vi "Write.vi"(8 "error in (no error)":errorcluster, 9 "Variant":variant, 10 "String":string, 11 "UDP in":refnum<class "UDP.lvclass">) -> (0 "error out":errorcluster, 3 "UDP out":refnum<class "UDP.lvclass">)   [LabVIEW 2019, in "Protocols.lvlib" / "UDP.lvclass"]
uses:
  UDP.lvclass
  UDP.lvclass/UDP.ctl
  Data Access/Read Target Port.vi
  Data Access/Read Target IP Address.vi
  Data Access/Read UDP Ref.vi
  Data Access/Write UDP Ref.vi
  <vilib>/Utility/error.llb/Clear Errors.vi
  Protocol Parent/Protocol Parent.lvclass
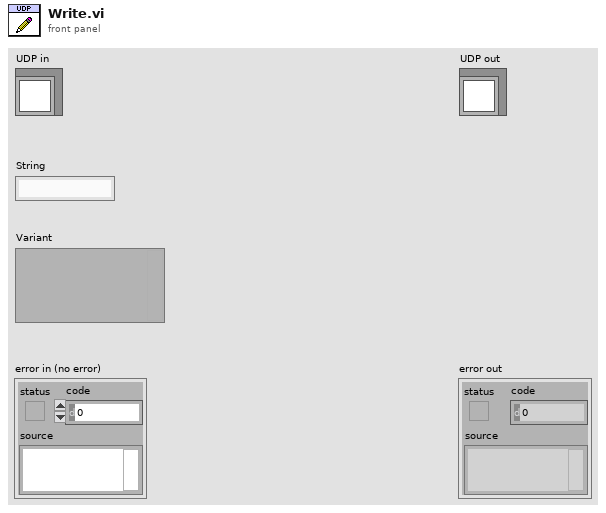
[diagram p1: front panel]
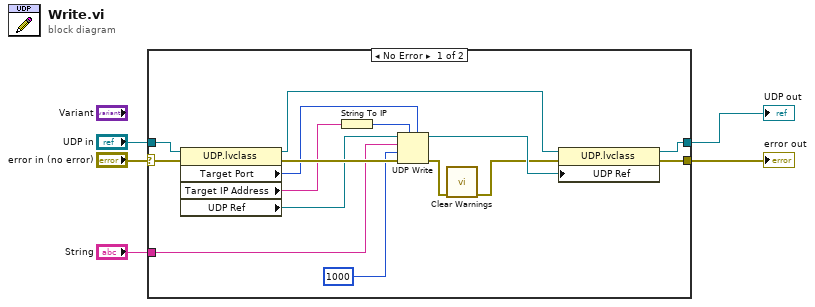
[diagram p0: block diagram]
diagram:
  n1 = case shown="No Error" "error in (no error)" {
    selector: "error in (no error)" -> [w13 w22]
    tunnel: "UDP in" -> [w19 w21]
    tunnel: [w16 w22] -> w5
    tunnel: [w15 w21] -> w4
    tunnel: "String" -> [w14 _]
    frame No Error {
      n2 = property class="UDP.lvclass"(reference=w19, error in=w13) -> (reference out=w18:refnum<class "UDP.lvclass">, error out=w20:errorcluster, "Target Port"=w11:u16, "Target IP Address"=w10:string, "UDP Ref"=w8:refnum<k16>)
      n3 = String To IP(1:w10) -> (0:w9:u32)
      n4 = UDP Write(address=w9, port or service name=w11, connection ID=w8, data in=w14, 8:w20, 9:1000 ("timeout ms (25000)")) -> (error out=w7:errorcluster, 3:w17:refnum<k16>)
      n5 = call "Clear Warnings.vi"("error in (no error)"=w7) -> ("error out"=w6:errorcluster)  [unwired: 10 in]
      n6 = property class="UDP.lvclass"(reference=w18, error in=w6, "UDP Ref"=w17) -> (reference out=w15:refnum<class "UDP.lvclass">, error out=w16:errorcluster)
    }
    frame Error {
    }
  }
  "error out" <- w5
  "UDP out" <- w4
